vi "main.vi"(8 "Error in":errorcluster) -> (0 "error out":errorcluster)   [LabVIEW 2018, in "User Console.lvlib"]
doc: "The main VI of the module."
uses:
  User Console.lvlib
  vi/Module Queue Actions.ctl
  ctl/Module State--enum.ctl
  Common/Common.lvlib
  Common/ctl/Stop all modules states--enum.ctl
  Error Handler/Error Handler.lvlib
  Error Handler/ctl/Module State--enum.ctl
  Error Handler/ctl/Error source--enum.ctl
  Common/ctl/Error to pass.ctl
  templates/ctl/Transactions--cluster.ctl
  Controller/Controller.lvlib
  Controller/ctl/Module State--enum.ctl
  ctl/Control references--cluster.ctl
  ctl/control enable states--cluster.ctl
  Controller/vi/state--global.vi
  templates/ctl/keypad--cluster.ctl
  templates/ctl/card reader--bool.ctl
panel:
  in  "Transactions":T1
  in  "Keypad":T2
  in  "Card Reader":T3
  # "User console"
  # "[Covers: UI1]"
  # "[Covers: UI2]"
  # "[Covers: UI2B]"
  # "[Covers: UI2C]"
  # "[Covers: ID1C]"
  # "[Covers: UI2A]"
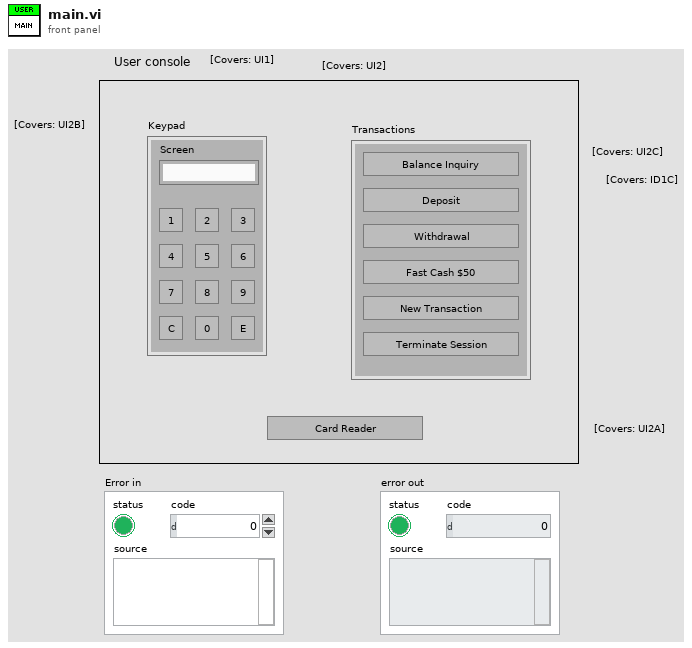
[diagram p1: front panel]
types:
  T1 = typedef "User Console.lvlib/Transactions--cluster.ctl" = cluster{"Balance Inquiry":bool, "Deposit":bool, "Withdrawal":bool, "Fast Cash $50":bool, "New Transaction":bool, "Terminate Session":bool}
  T2 = typedef "User Console.lvlib/keypad--cluster.ctl" = cluster{"Screen":string, "1":bool, "2":bool, "3":bool, "4":bool, "5":bool, "6":bool, "7":bool, "8":bool, "9":bool, "C":bool, "0":bool, "E":bool}
  T3 = typedef "User Console.lvlib/card reader--bool.ctl" = bool
  T4 = typedef "User Console.lvlib/Control references--cluster.ctl" = cluster{"Transactions":refnum<vi>, "Card Reader":refnum<vi>, "Keypad":refnum<vi>}
  T5 = typedef "User Console.lvlib/Module Queue Actions.ctl" = enum16{"Create", "Get", "Destroy"}
  T6 = typedef "Common.lvlib/Stop all modules states--enum.ctl" = enum16{"Create", "Get", "Send 'Stop all' Message", "Destroy"}
  T7 = typedef "User Console.lvlib/Module State--enum.ctl" = enum16{"Init", "Error", "Idle", "Close", "Transaction Button Pressed: Which?", "Balance Inquiry Pressed", "Desposit Pressed", "Withdrawal Pressed", "Fast Cash Pressed", "New Transaction Pressed", "Terminate Session Pressed", "Card Reader Pressed", "Keypad Button Pressed", "Update Keypad Screen", "Enable/disable controls", "Card reader: On?"}
  T8 = typedef "Common.lvlib/Error source--enum.ctl" = enum16{"Display Console", "User Console", "Sensor Interface IO", "Process Step", "Other"}
  T9 = typedef "Common.lvlib/Error to pass.ctl" = cluster{"Error source":T8, "Error":errorcluster}
  T10 = typedef "Error Handler.lvlib/Module State--enum.ctl" = enum16{"Init", "Error", "Idle", "Close", "Handle External Error", "Log to file"}
  T11 = typedef "Controller.lvlib/Module State--enum.ctl" = enum16{"Init", "Error", "Close", "User Console: Card Reader Pressed", "Sensor Interface: Deposit Received pressed", "Sensor Interface: Funds Dispensed Pressed", "Idle", "Login State", "Balance Enquiry", "Deposit State", "Withdrawal State", "Fast Cash State", "Configuration Database", "Inactivity Timeout", "Terminate State", "Wait for account number", "Verify account number", "Wait for new transaction button"}
  T12 = typedef "User Console.lvlib/control enable states--cluster.ctl" = cluster{"Transactions":enum8{"Enabled", "Disabled", "Disabled and Grayed Out"}, "Card reader":enum8{"Enabled", "Disabled", "Disabled and Grayed Out"}, "Keypad":enum8{"Enabled", "Disabled", "Disabled and Grayed Out"}}
  T13 = enum8{"Enabled", "Disabled", "Disabled and Grayed Out"}
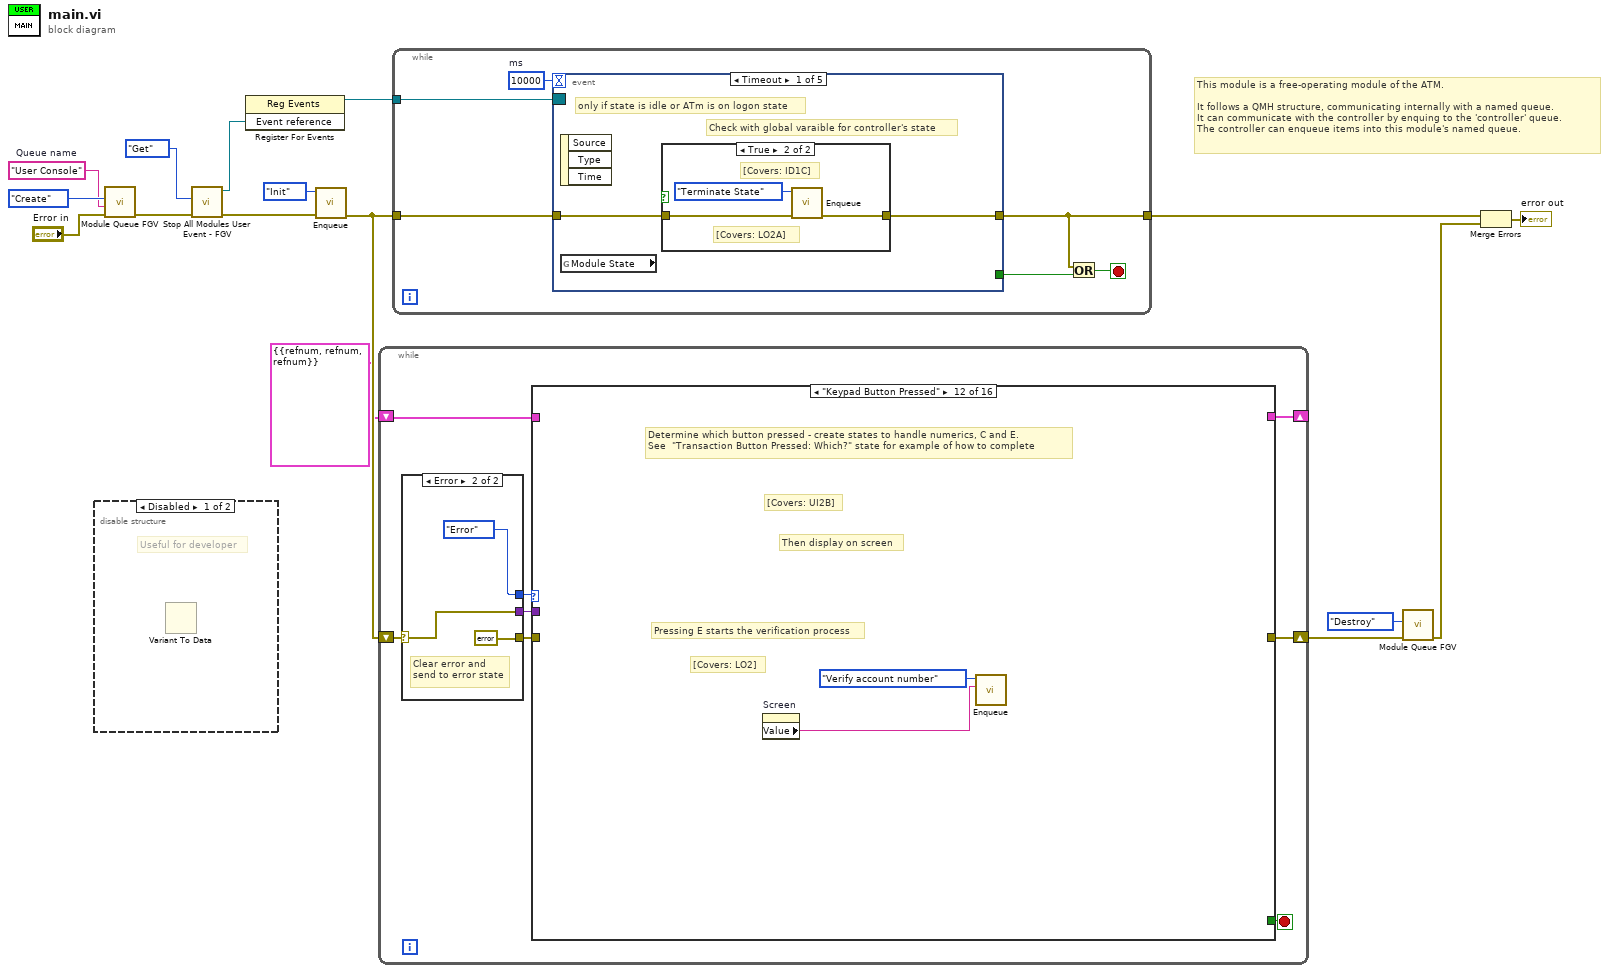
[diagram p0: block diagram]
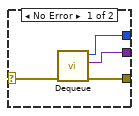
[diagram p3: hidden frame]
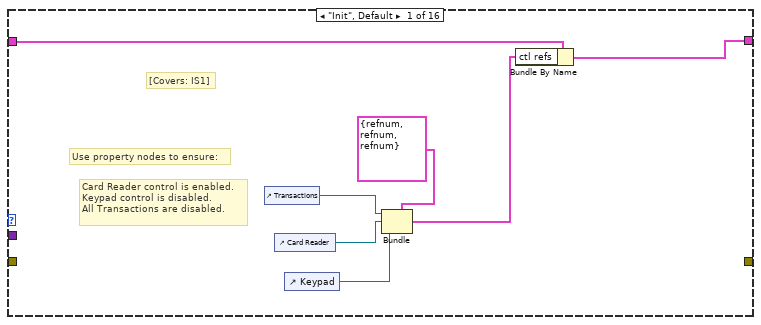
[diagram p4: hidden frame]
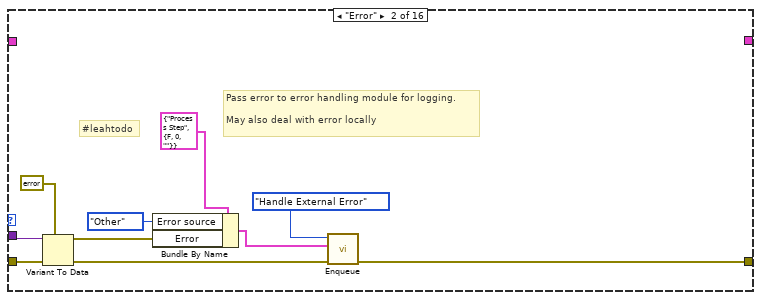
[diagram p5: hidden frame]
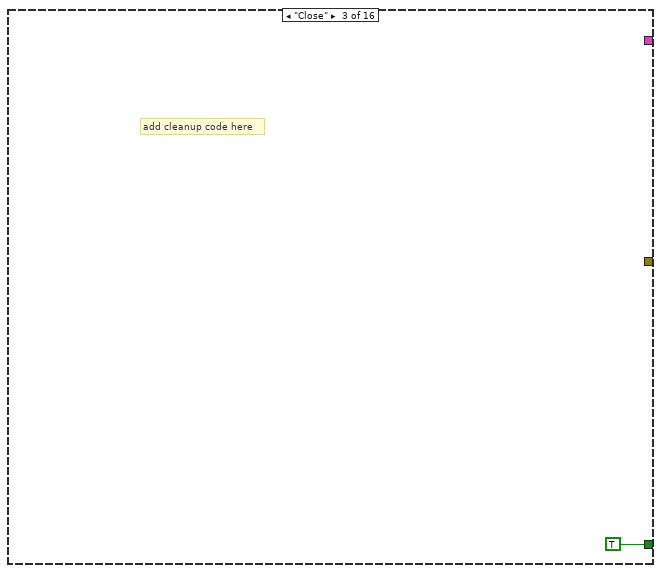
[diagram p6: hidden frame]
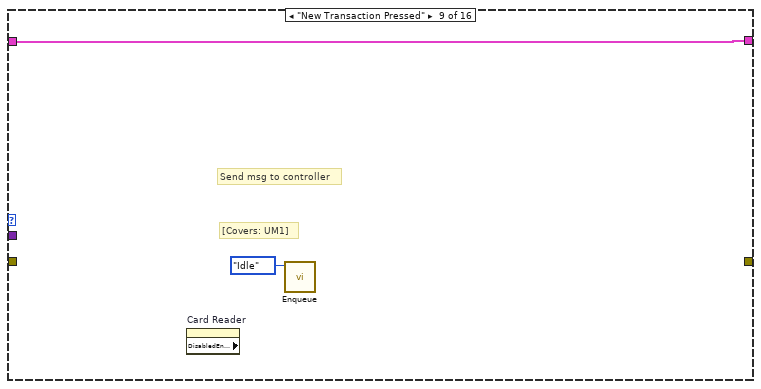
[diagram p12: hidden frame]
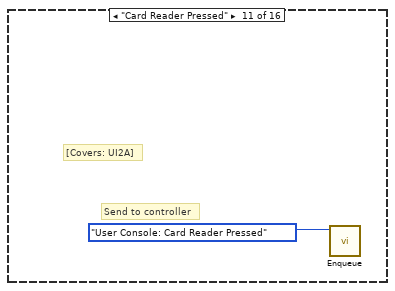
[diagram p14: hidden frame]
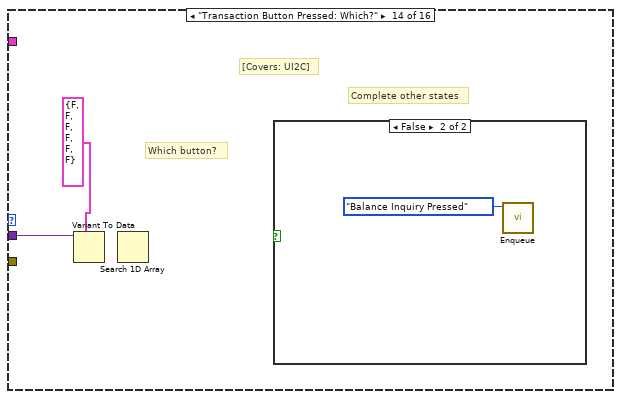
[diagram p16: hidden frame]
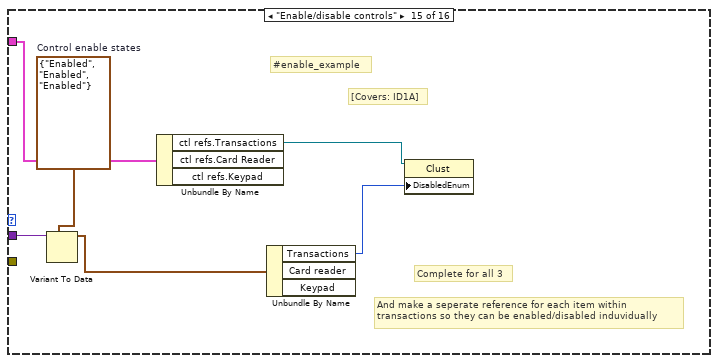
[diagram p18: hidden frame]
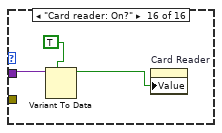
[diagram p19: hidden frame]
diagram:
  w15 = "User Console"  # Queue name
  # "This module is a free-operating module of the ATM.\n\nIt follows a QMH structure, communicating internally with a named queue.\nIt can communicate with the controller by enquing to the 'controller' queue.\nThe controller can enqueue items into this module's named queue."
  n1 = disable-structure shown="Disabled" {
    frame Disabled {
      # "Useful for developer"
      n2 = Variant To Data() -> ()  [unwired: 3 in, 2 out]
    }
    frame Enabled {
    }
  }
  n3 = call "Module Queue FGV.vi"("Error in"="Error in", "Queue name"=w15, "Module Queue Actions"=Module_Queue_Actions."Create") -> ("error out"=w10:errorcluster)  [unwired: 7 in, 1 out]
  n4 = call "Stop All Modules User Event - FGV.vi"("error in"=w10, "Action"=Stop_all_modules_states--enum."Get") -> ("error out"=w9:errorcluster, "Event reference"=w12:refnum<user-event>)  [unwired: 8 in]
  n5 = register-events(w12) -> (reference out=w11:refnum<event-registration>)  [unwired: 2 in, 1 out]
  n6 = call "Enqueue.vi"("error in (no error)"=w9, "State"=Module_State--enum."Init") -> ("error out"=w8:errorcluster)  [unwired: 9 in]
  n7 = while {
    shift-right: [w21] -> w6
    shift-left: w8 -> [w20]
    shift-right: [w17] -> _
    shift-left: cluster{"ctl refs":T4} {"ctl refs"={"Transactions"=refnum, "Card Reader"=refnum, "Keypad"=refnum}} -> [w18]
    stop <- w19 stop-if-true
    n8 = case shown="Error" w20 {
      selector: w20 -> [w25 w30]
      tunnel: [w28 Module_State--enum."Error" ("State")] -> w24
      tunnel: [w27 w30] -> w23
      tunnel: [w26 errorcluster {"status"=FALSE, "code"=0, "source"=""} ("error out")] -> w22
      frame No Error {
        n9 = call "Dequeue.vi"("error in (no error)"=w25) -> ("error out"=w26:errorcluster, "Data"=w27:variant, "State"=w28:T7)  [unwired: 8 in]
      }
      frame Error {
        # "Clear error and\nsend to error state"
      }
    }
    n10 = case shown="\"Keypad Button Pressed\"" w24 {
      tunnel: w23 -> [_ w45 _ _ _ _ _ _ _ _ _ _ _ w56 w58 w64]
      tunnel: w22 -> [_ w46 _ _ _ _ _ _ _ _ _ _ _ _ _ _]
      tunnel: [_ w47 _ _ _ _ _ _ _ _ _ _ _ _ _ _] -> w21
      tunnel: [_ _ TRUE _ _ _ _ _ _ _ _ _ _ _ _ _] -> w19
      tunnel: w18 -> [w33 _ _ _ _ _ _ _ w50 _ _ _ _ _ w63 _]
      tunnel: [w34 _ _ _ _ _ _ _ w50 _ _ _ _ _ _ _] -> w17
      frame "Init", Default {
        # "Use property nodes to ensure:"
        # "Card Reader control is enabled.\nKeypad control is disabled.\nAll Transactions are disabled."
        # "[Covers: IS1]"
        n11 = control-ref of="Transactions"() -> (w36:refnum<vi>)
        n12 = control-ref of="Card Reader"() -> (w37:refnum<vi>)
        n13 = control-ref of="Keypad"() -> (w38:refnum<vi>)
        n14 = Bundle(cluster=T4 {"Transactions"=refnum, "Card Reader"=refnum, "Keypad"=refnum} ("output cluster"), "Transactions"=w36, "Card Reader"=w37, "Keypad"=w38) -> (w32:T4)
        n15 = Bundle By Name(cluster=w33, "ctl refs"=w32) -> (w34:cluster{"ctl refs":T4})
      }
      frame "Error" {
        # "#leahtodo"
        # "Pass error to error handling module for logging.\n\nMay also deal with error locally"
        n16 = Variant To Data(error in=w46, type=errorcluster {"status"=FALSE, "code"=0, "source"=""} ("error constant"), Variant=w45) -> (data=w41:errorcluster, error out=w43:errorcluster)
        n17 = Bundle By Name(cluster=T9 {"Error source"=enum."Process Step", "Error"={"status"=FALSE, "code"=0, "source"=""}} ("Error to pass"), "Error source"=Error_source--enum."Other", "Error"=w41) -> (w40:T9)
        n18 = call "Enqueue.vi"("error in (no error)"=w43, "Data"=w40, "State"=Module_State--enum."Handle External Error") -> ("error out"=w47:errorcluster)  [unwired: 8 in]
      }
      frame "Close" {
        # "add cleanup code here"
      }
      frame "Idle" {
      }
      frame "Balance Inquiry Pressed" {
      }
      frame "Desposit Pressed" {
      }
      frame "Withdrawal Pressed" {
      }
      frame "Fast Cash Pressed" {
      }
      frame "New Transaction Pressed" {
        # "Send msg to controller"
        # "[Covers: UM1]"
        n19 = property on="Card Reader" class="Bool" props=["DisabledEnum"]() -> ()  [unwired: 2 in, 3 out]
        n20 = call "Enqueue.vi"("State"=Module_State--enum."Idle") -> ()  [unwired: 10 in, 1 out]
      }
      frame "Terminate Session Pressed" {
      }
      frame "Card Reader Pressed" {
        # "Send to controller"
        # "[Covers: UI2A]"
        n21 = call "Enqueue.vi"("State"=Module_State--enum."User Console: Card Reader Pressed") -> ()  [unwired: 10 in, 1 out]
      }
      frame "Keypad Button Pressed" {
        # "[Covers: LO2]"
        # "Pressing E starts the verification process"
        # "Then display on screen"
        # "[Covers: UI2B]"
        # "Determine which button pressed - create states to handle numerics, C and E.\nSee  \"Transaction Button Pressed: Which?\" state for example of how to complete"
        n22 = property on="Screen" class="Str"() -> ("Value"=w53:string)  [unwired: 2 in, 2 out]
        n23 = call "Enqueue.vi"("Data"=w53, "State"=Module_State--enum."Verify account number") -> ()  [unwired: 9 in, 1 out]
      }
      frame "Update Keypad Screen" {
      }
      frame "Transaction Button Pressed: Which?" {
        # "[Covers: UI2C]"
        # "Complete other states"
        # "Which button?"
        n24 = Variant To Data(type=T1 {"Balance Inquiry"=FALSE, "Deposit"=FALSE, "Withdrawal"=FALSE, "Fast Cash $50"=FALSE, "New Transaction"=FALSE, "Terminate Session"=FALSE} ("NewVal"), Variant=w56) -> ()  [unwired: 1 in, 2 out]
        n25 = Search 1D Array() -> ()  [unwired: 3 in, 1 out]
        n26 = case shown="\"Balance Enquiry Pressed\"" {
          selector: _ -> [_ _]
          frame False {
          }
          frame False {
            n27 = call "Enqueue.vi"("State"=Module_State--enum."Balance Inquiry Pressed") -> ()  [unwired: 10 in, 1 out]
          }
        }
      }
      frame "Enable/disable controls" {
        w60 = T12 {"Transactions"=enum."Enabled", "Card reader"=enum."Enabled", "Keypad"=enum."Enabled"}  # Control enable states
        # "And make a seperate reference for each item within\ntransactions so they can be enabled/disabled induvidually"
        # "#enable_example"
        # "[Covers: ID1A]"
        # "Complete for all 3"
        n28 = Variant To Data(type=w60, Variant=w58) -> (data=w59:T12)  [unwired: 1 in, 1 out]
        n29 = Unbundle By Name(w63) -> ("ctl refs.Transactions"=w62:refnum<vi>)  [unwired: 2 out]
        n30 = Unbundle By Name(w59) -> ("Transactions"=w61:T13)  [unwired: 2 out]
        n31 = property class="Clust"(reference=w62, "DisabledEnum"=w61) -> ()  [unwired: 1 in, 2 out]
      }
      frame "Card reader: On?" {
        n32 = Variant To Data(type=TRUE, Variant=w64) -> (data=w66:bool)  [unwired: 1 in, 1 out]
        n33 = property on="Card Reader" class="Bool"("Value"=w66) -> ()  [unwired: 2 in, 2 out]
      }
    }
  }
  n34 = while {
    tunnel: w8 -> [w72]
    tunnel: [w69] -> w4
    tunnel: w11 -> [w71]
    stop <- w70 stop-if-true
    w67 = 10000  # ms
    n35 = event shown="[0] Timeout" {
      selector: w71 -> [_ _ _ _ _]
      dyn-events: _ -> [_ _ _ _ _]
      timeout: w67 -> [_ _ _ _ _]
      tunnel: w72 -> [w74 w81 _ w86 w89]
      tunnel: [w73 w80 _ w85 w90] -> w69
      tunnel: [_ TRUE _ _ _] -> w68
      event Timeout {
        # "Check with global varaible for controller's state"
        # "only if state is idle or ATm is on logon state"
        n36 = event-data() -> ()  [unwired: 1 in, 3 out]
        n37 = global read "state--global.vi" "Module State"() -> ()  [unwired: 1 out]
        n38 = case shown="True" {
          selector: _ -> [_ _]
          tunnel: w74 -> [_ w76]
          tunnel: [_ w75] -> w73
          frame False {
          }
          frame True {
            # "[Covers: LO2A]"
            # "[Covers: ID1C]"
            n39 = call "Enqueue.vi"("error in (no error)"=w76, "State"=Module_State--enum."Terminate State") -> ("error out"=w75:errorcluster)  [unwired: 9 in]
          }
        }
      }
      event User Event {
        # "Stop message has been received - shut down"
        n40 = event-data() -> ()  [unwired: 1 in, 1 out]
        n41 = call "Enqueue.vi"("error in (no error)"=w81, "State"=Module_State--enum."Close") -> ("error out"=w80:errorcluster)  [unwired: 9 in]
      }
      event Value Change {
        n42 = event-data() -> ("NewVal"=w82:T2)  [unwired: 1 in, 5 out]
        n43 = call "Enqueue.vi"("Data"=w82, "State"=Module_State--enum."Keypad Button Pressed") -> ()  [unwired: 9 in, 1 out]
      }
      event Value Change {
        n44 = event-data() -> ("NewVal"=w84:T1)  [unwired: 1 in]
        n45 = call "Enqueue.vi"("error in (no error)"=w86, "Data"=w84, "State"=Module_State--enum."Transaction Button Pressed: Which?") -> ("error out"=w85:errorcluster)  [unwired: 8 in]
      }
      event Value Change {
        n46 = event-data() -> ()  [unwired: 1 in, 6 out]
        n47 = call "Enqueue.vi"("error in (no error)"=w89, "State"=Module_State--enum."Card Reader Pressed") -> ("error out"=w90:errorcluster)  [unwired: 9 in]
      }
    }
    n48 = Or(x=w69, y=w68) -> (x .or. y?=w70:bool)
  }
  n49 = call "Module Queue FGV.vi"("Error in"=w6, "Module Queue Actions"=Module_Queue_Actions."Destroy") -> ("error out"=w5:errorcluster)  [unwired: 8 in, 1 out]
  n50 = Merge Errors(w4, w5) -> (→"error out":errorcluster)
